vi "Flash Drive Error Conn Message.vi"() -> ()   [LabVIEW 2018]
panel:
  in  "OK":bool
  # "Flash Drive Connection Issue"
  # "Cannot connect to the Flash Directory on the cRIO:\n1) Make sure a fat32 formatted flash drive is inserted into the cRIO.\n\n2) Make sure the cRIO is mapped as a network drive on the main PC (see fig.1 below).  Webdav needs to be installed on the cRIO in order to do this. \n\n3) Make sure the correct path is entered in the Rig Config Settings for \"cRIO Test Data Dir\".  The flash drive will always be \"u\".  So, if the cRIO is mapped as network drive U then the correct path to put in the Rig Config Settings would be \"U:\\u\".\n\n4) Make sure the mapped network drive path is connected (figure 1).  If it isn't you will have to double click on the path at which point a login window will pop up.  Enter your Admin login and password.  If you do not have one then create one on the cRIO using via the \"Web Configuration\" page.  The default login for the cRIO is:   User name:  \"admin\"\n                                                                    Password:  blank"
  # "Figure 1 - cRIO Mapped Network Drive"
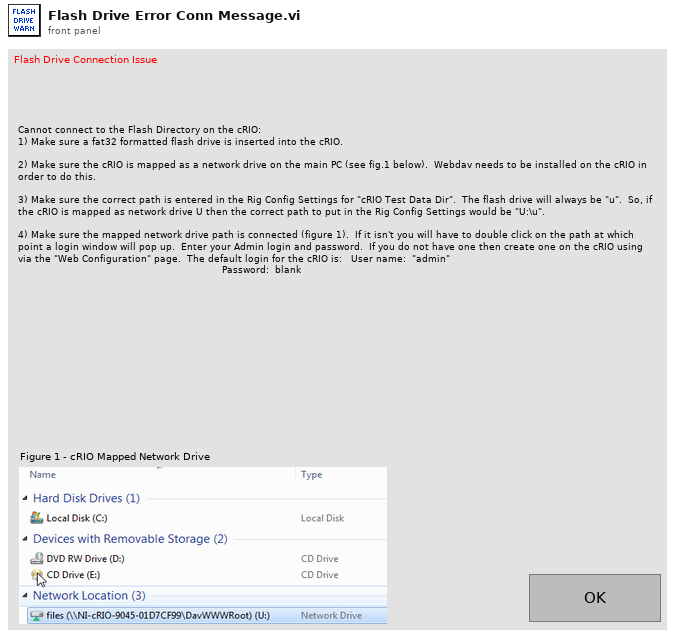
[diagram p1: front panel]
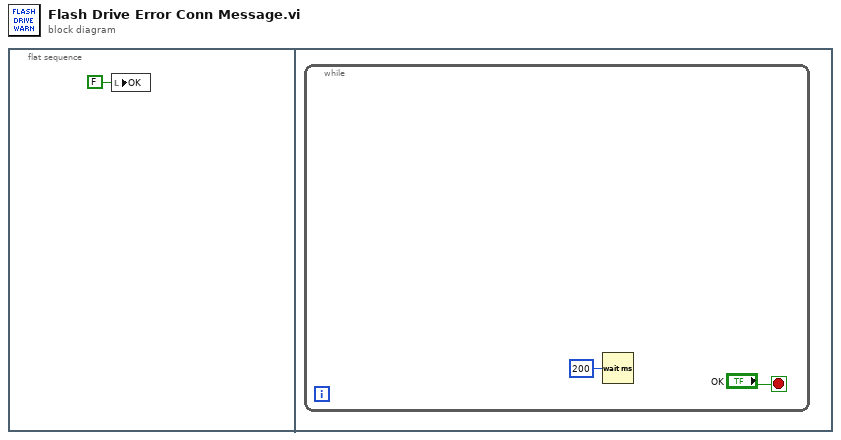
[diagram p0: block diagram]
diagram:
  n1 = flat-sequence {
    frame #0 {
      n2 = local write "OK"(FALSE ("OK")) -> ()
    }
    frame #1 {
      n3 = while {
        stop <- "OK" stop-if-true
        n4 = Wait (ms)(milliseconds to wait=u32 200) -> ()  [unwired: 1 out]
      }
    }
  }
